vi "SRS -- publish -- handle.vi"(7 "publisher action":T1, 9 "SRS865 visa":refnum<visa-resource-name>) -> (1 "SRS865 visa OUT":refnum<visa-resource-name>)   [LabVIEW 2018]
uses:
  publisher action.ctl
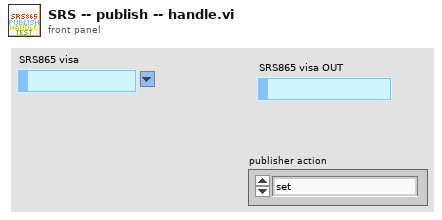
[diagram p1: front panel]
types:
  T1 = typedef "publisher action.ctl" = enum16{"set", "get", "init", "check"}
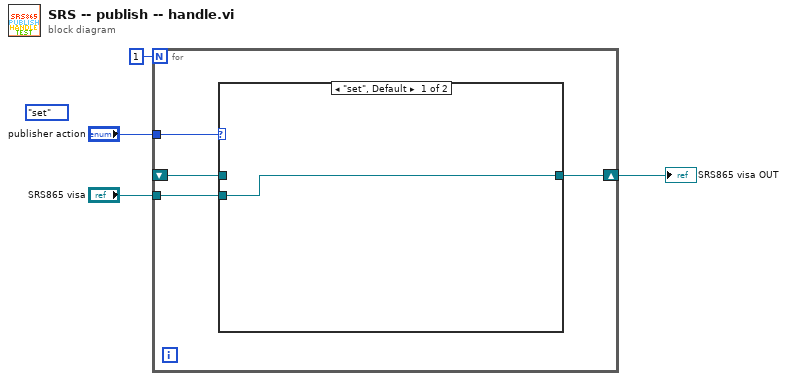
[diagram p0: block diagram]
diagram:
  (unwired) publisher_action."set" ("publisher action")
  n1 = for {
    N: 1 -> [_]
    tunnel: "publisher action" -> [w8]
    tunnel: "SRS865 visa" -> [w6]
    shift-right: [w7] -> w2
    shift-left: _ -> [w5]
    n2 = case shown="\"set\", Default" w8 {
      tunnel: [w9 w10] -> w7
      tunnel: w6 -> [w9 _]
      tunnel: w5 -> [_ w10]
      frame "set", Default {
      }
      frame "get" {
      }
    }
  }
  "SRS865 visa OUT" <- w2
